vi "NIIE_Layer_View.vi"(7 "Add To Undo?":bool, 8 "Error":errorcluster, 11 "Data":T1={"Class"={"Ants"=refnum, "Layer"=refnum, "Templates"=refnum, "Icon"=refnum, "Glyph"=refnum, "Settings"=refnum, "Tools"=refnum}, "Ref"={"Add Layer"=refnum, "Remove Layer"=refnum, "Line Text"=[], "Body Text Spec"=refnum, "DNL_Font"=refnum, "glyph path str"=refnum, "templates path str"=refnum, "Arrow Up"=refnum, "Arrow Down"=refnum, "IE VI Ref"=refnum, "Glyphs tree"=refnum, "Templates tree"=refnum, "Layer Icon Text"=refnum, "Layer Template"=refnum, "Clipboard"=refnum, "BW icon in"=refnum, "Color icon in"=refnum, "Layer Clust"=refnum, "Body Text"=refnum, "DNL_Framework Templates"=refnum, "Search Templates"=refnum, "TextMarker"=refnum, "Tab Control"=refnum, "Search Glyphs"=refnum, "Line Color"=refnum, "DNL_Glyphs []"=refnum, "Fill Color"=refnum, "Tools"=refnum, "Glyphs tree"=refnum, "Icon"=refnum, "Preview"=refnum, "Ants"=refnum, "Terminals"=refnum, "menu reference"=refnum, "LayerNames"=[], "GlyphLoadAnimation"=refnum, "TemplateLoadAnimation"=refnum, "refreshGlyphs"=refnum, "refreshTemplates"=refnum}, "Support"={"AntsRect"={"left"=0, "top"=0, "right"=0, "bottom"=0}, "Mouse Move Coords"={"Horizontal"=0, "Vertical"=0}, "Mouse Down Coords"={"Horizontal"=0, "Vertical"=0}, "Temp Coord"={"Horizontal"=0, "Vertical"=0}, "Action"=enum."Default", "Edge Color"=4914962, "Fill Color"=16860, "Mouse Down?"=FALSE, "Draft Mode?"=FALSE, "Temp Icon"=bytes[3102], "CTRL Pressed"=FALSE, "Move Selection?"=FALSE, "AntsRect Orig"={"left"=0, "top"=0, "right"=0, "bottom"=0}, "Text"="", "TM Set?"=FALSE, "Mouse inside icon?"=FALSE, "Tool (old value)"=0, "Pencil Move Color"=0, "Swap Colors?"=FALSE, "Shift pressed?"=FALSE}}) -> (0 "Error Out":errorcluster, 3 "Data Out":T1={"Class"={"Ants"=refnum, "Layer"=refnum, "Templates"=refnum, "Icon"=refnum, "Glyph"=refnum, "Settings"=refnum, "Tools"=refnum}, "Ref"={"Add Layer"=refnum, "Remove Layer"=refnum, "Line Text"=[], "Body Text Spec"=refnum, "DNL_Font"=refnum, "glyph path str"=refnum, "templates path str"=refnum, "Arrow Up"=refnum, "Arrow Down"=refnum, "IE VI Ref"=refnum, "Glyphs tree"=refnum, "Templates tree"=refnum, "Layer Icon Text"=refnum, "Layer Template"=refnum, "Clipboard"=refnum, "BW icon in"=refnum, "Color icon in"=refnum, "Layer Clust"=refnum, "Body Text"=refnum, "DNL_Framework Templates"=refnum, "Search Templates"=refnum, "TextMarker"=refnum, "Tab Control"=refnum, "Search Glyphs"=refnum, "Line Color"=refnum, "DNL_Glyphs []"=refnum, "Fill Color"=refnum, "Tools"=refnum, "Glyphs tree"=refnum, "Icon"=refnum, "Preview"=refnum, "Ants"=refnum, "Terminals"=refnum, "menu reference"=refnum, "LayerNames"=[], "GlyphLoadAnimation"=refnum, "TemplateLoadAnimation"=refnum, "refreshGlyphs"=refnum, "refreshTemplates"=refnum}, "Support"={"AntsRect"={"left"=0, "top"=0, "right"=0, "bottom"=0}, "Mouse Move Coords"={"Horizontal"=0, "Vertical"=0}, "Mouse Down Coords"={"Horizontal"=0, "Vertical"=0}, "Temp Coord"={"Horizontal"=0, "Vertical"=0}, "Action"=enum."Default", "Edge Color"=4914962, "Fill Color"=16860, "Mouse Down?"=FALSE, "Draft Mode?"=FALSE, "Temp Icon"=bytes[3102], "CTRL Pressed"=FALSE, "Move Selection?"=FALSE, "AntsRect Orig"={"left"=0, "top"=0, "right"=0, "bottom"=0}, "Text"="", "TM Set?"=FALSE, "Mouse inside icon?"=FALSE, "Tool (old value)"=0, "Pencil Move Color"=0, "Swap Colors?"=FALSE, "Shift pressed?"=FALSE}})   [LabVIEW 2021]
uses:
  Controls/IE Data.ctl
  Class/Ants/Ants.lvclass
  Class/FakedArray/FakedArray.lvclass
  Class/Icon Library/Glyph.lvclass
  Class/Settings/Settings.lvclass
  Class/Tools/Tools Paint.lvclass
  vi.lib/LabVIEW Icon API/lv_icon/Classes/Icon/Icon.lvclass
  Controls/IE Classes.ctl
  Controls/References Cluster.ctl
  Controls/SupportClass.ctl
  <vilib>/Utility/miscctls.llb/LVPoint32TypeDef.ctl
  Controls/ENUM_SupportClass_Action.ctl
  vi.lib/LabVIEW Icon API/lv_icon/Controls/IEColor.ctl
  vi.lib/LabVIEW Icon API/lv_icon/Classes/Layer/Layer.lvclass
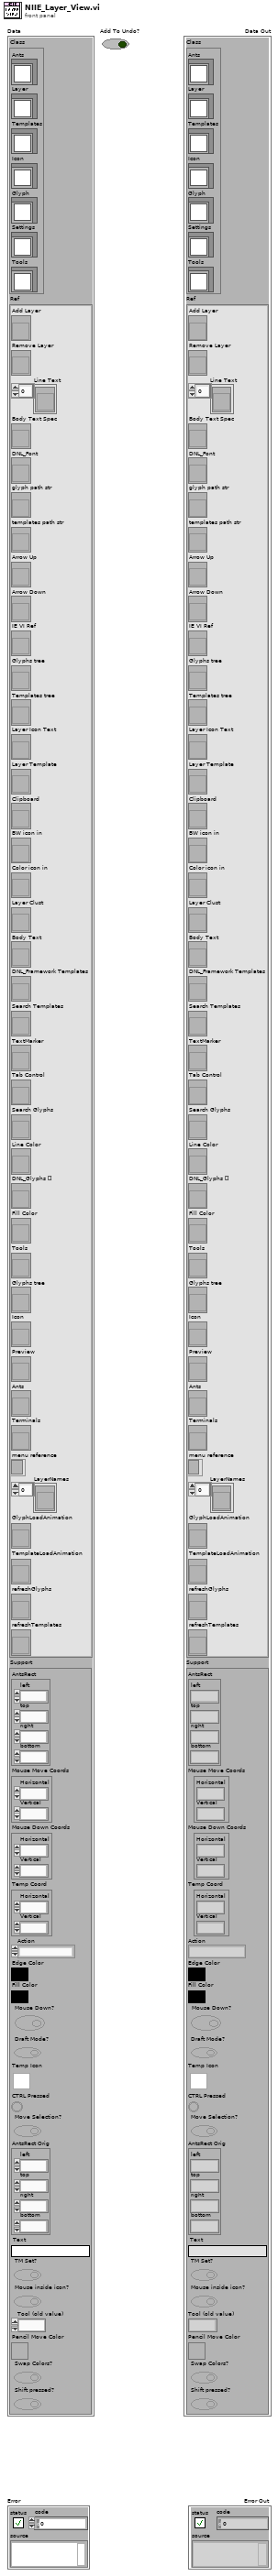
[diagram p1: front panel]
types:
  T1 = typedef "IE Data.ctl" = cluster{"Class":T2, "Ref":T3, "Support":T4}
  T2 = typedef "IE Classes.ctl" = cluster{"Ants":refnum<class "Ants.lvclass">, "Layer":refnum<class "FakedArray.lvclass">, "Templates":refnum<class "FakedArray.lvclass">, "Icon":refnum<class "Icon.lvclass">, "Glyph":refnum<class "Glyph.lvclass">, "Settings":refnum<class "Settings.lvclass">, "Tools":refnum<class "Tools Paint.lvclass">}
  T3 = typedef "References Cluster.ctl" = cluster{"Add Layer":refnum<vi>, "Remove Layer":refnum<vi>, "Line Text":refnum<vi>[], "Body Text Spec":refnum<vi>, "DNL_Font":refnum<vi>, "glyph path str":refnum<vi>, "templates path str":refnum<vi>, "Arrow Up":refnum<vi>, "Arrow Down":refnum<vi>, "IE VI Ref":refnum<vi>, "Glyphs tree":refnum<vi>, "Templates tree":refnum<vi>, "Layer Icon Text":refnum<vi>, "Layer Template":refnum<vi>, "Clipboard":refnum<vi>, "BW icon in":refnum<vi>, "Color icon in":refnum<vi>, "Layer Clust":refnum<vi>, "Body Text":refnum<vi>, "DNL_Framework Templates":refnum<vi>, "Search Templates":refnum<vi>, "TextMarker":refnum<vi>, "Tab Control":refnum<vi>, "Search Glyphs":refnum<vi>, "Line Color":refnum<vi>, "DNL_Glyphs []":refnum<vi>, "Fill Color":refnum<vi>, "Tools":refnum<vi>, "Glyphs tree":refnum<vi>, "Icon":refnum<vi>, "Preview":refnum<vi>, "Ants":refnum<vi>, "Terminals":refnum<vi>, "menu reference":refnum<k9>, "LayerNames":refnum<vi>[], "GlyphLoadAnimation":refnum<vi>, "TemplateLoadAnimation":refnum<vi>, "refreshGlyphs":refnum<vi>, "refreshTemplates":refnum<vi>}
  T4 = typedef "SupportClass.ctl" = cluster{"AntsRect":cluster{"left":i16, "top":i16, "right":i16, "bottom":i16}, "Mouse Move Coords":T5, "Mouse Down Coords":T5, "Temp Coord":T5, "Action":T6, "Edge Color":T7, "Fill Color":T7, "Mouse Down?":bool, "Draft Mode?":bool, "Temp Icon":picture, "CTRL Pressed":bool, "Move Selection?":bool, "AntsRect Orig":cluster{"left":i16, "top":i16, "right":i16, "bottom":i16}, "Text":string, "TM Set?":bool, "Mouse inside icon?":bool, "Tool (old value)":u32, "Pencil Move Color":u32, "Swap Colors?":bool, "Shift pressed?":bool}
  T5 = typedef "LVPoint32TypeDef.ctl" = cluster{"Horizontal":i32, "Vertical":i32}
  T6 = typedef "ENUM_SupportClass_Action.ctl" = enum16{"Default", "Move Selection", "Glyph Library", "Tool"}
  T7 = typedef "IEColor.ctl" = u32
  T8 = cluster{"Pointer Absolute":i32, "Cluster Refnum":refnum<vi>, "# Rows":i32, "# Cols":i32, "Scrollbar Position":i32, "Pointer Absolute Row":i32, "Pointer Absolute Col":i32}
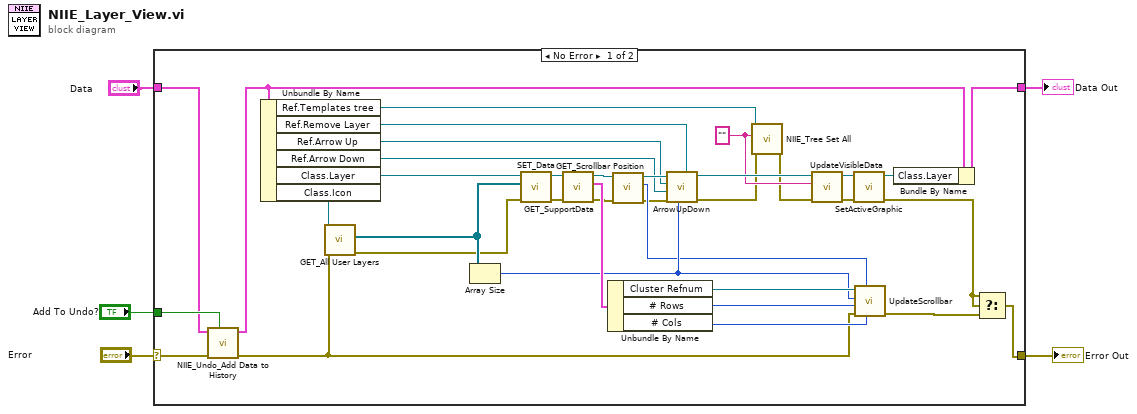
[diagram p0: block diagram]
diagram:
  n1 = case shown="No Error" "Error" {
    selector: "Error" -> [w41 w43]
    tunnel: [w23 w43] -> w4
    tunnel: "Add To Undo?" -> [w40 _]
    tunnel: "Data" -> [w19 w42]
    tunnel: [w20 w42] -> w1
    frame No Error {
      w8 = "" ("Value")
      n2 = call "NIIE_Undo_Add Data to History.vi"("Add To Undo?"=w40, "Error"=w41, "Data"=w19) -> ("Error Out"=w15:errorcluster, "Data Out"=w18:T1)  [unwired: 7 out]
      n3 = Unbundle By Name(w18) -> ("Ref.Templates tree"=w9:refnum<vi>, "Ref.Remove Layer"=w10:refnum<vi>, "Ref.Arrow Up"=w11:refnum<vi>, "Ref.Arrow Down"=w12:refnum<vi>, "Class.Layer"=w22:refnum<class "FakedArray.lvclass">, "Class.Icon"=w17:refnum<class "Icon.lvclass">)
      n4 = call-dynamic "GET_All User Layers.vi"("error in (no error)"=w15, "Icon.lvclass in"=w17) -> ("error out"=w14:errorcluster, "User Layer"=w16:refnum<class "Layer.lvclass">[])  [unwired: 8 out]
      n5 = Array Size(array=w16) -> (size(s)=w31:i32)
      n6 = call-dynamic "SET_Data.vi"("Error"=w14, "Data"=w16, "FakedArray"=w22) -> ("Error Out"=w33:errorcluster, "FakedArray Out"=w32:refnum<class "FakedArray.lvclass">)  [unwired: 7 out]
      n7 = call-dynamic "GET_SupportData.vi"("error in (no error)"=w33, "FakedArray in"=w32) -> ("error out"=w30:errorcluster, "Cluster"=w34:T8, "FakedArray out"=w29:refnum<class "FakedArray.lvclass">)  [unwired: 7 out]
      n8 = Unbundle By Name(w34) -> ("Cluster Refnum"=w35:refnum<vi>, "# Rows"=w36:i32, "# Cols"=w27:i32)
      n9 = call-dynamic "GET_Scrollbar Position.vi"("error in (no error)"=w30, "FakedArray.lvclass in"=w29) -> ("error out"=w26:errorcluster, "Scrollbar Position"=w28:i32, "FakedArray.lvclass out"=w25:refnum<class "FakedArray.lvclass">)  [unwired: 7 out]
      n10 = call "ArrowUpDown.vi"("Remove Layer"=w10, "# Layers"=w31, "Error"=w26, "Arrow Down"=w12, "Arrow Up"=w11, "FakedArray"=w25) -> ("Error Out"=w7:errorcluster, "FakedArray Out"=w37:refnum<class "FakedArray.lvclass">)  [unwired: 4 out]
      n11 = call "NIIE_Tree Set All.vi"("Error"=w7, "Value"=w8, "TreeControl"=w9) -> ("Error Out"=w6:errorcluster)  [unwired: 7 in, 1 out]
      n12 = call-dynamic "UpdateVisibleData.vi"("Error"=w6, "Keyword"=w8, "FakedArray"=w37) -> ("Error Out"=w38:errorcluster, "FakedArray Out"=w39:refnum<class "FakedArray.lvclass">)  [unwired: 2 in, 5 out]
      n13 = call-dynamic "SetActiveGraphic.vi"("error in (no error)"=w38, "FakedArray in"=w39) -> ("error out"=w13:errorcluster, "FakedArray out"=w21:refnum<class "FakedArray.lvclass">)  [unwired: 4 in, 4 out]
      n14 = call "UpdateScrollbar.vi"("# Cols"=w27, "Value Scrollbar"=w28, "error in"=w15, "#Rows"=w36, "# Elements"=w31, "Cluster Refnum"=w35) -> ("error out"=w24:errorcluster)  [unwired: 5 out]
      n15 = Bundle By Name(cluster=w18, "Class.Layer"=w21) -> (w20:T1)
      n16 = Select(t=w13, s=w13, f=w24) -> (s? t:f=w23:errorcluster)
    }
    frame Error {
    }
  }
  "Error Out" <- w4
  "Data Out" <- w1
